vi "Corr Digitizer Save INFO.vi"(7 "path template":path, 8 "error in":errorcluster, 9 "digitizer info":T2, 10 "correction type":T1, 11 "path result":path) -> (0 "error out":errorcluster)   [LabVIEW 2013]
doc: "Saves digitizer/channel INFO file."
uses:
  Corr Digitizer INFO.ctl
  Corr Digitizer INFO item.ctl
  Corr Digitizer INFO parameter.ctl
  Corr CSV Template.ctl
  Corr Digitizer Type.ctl
  octave/infolib.lvlibp/Private/Add key polymorph parts/String.vi
  octave/infolib.lvlibp/Private/Add matrix polymorph parts/1D String.vi
  octave/infolib.lvlibp/Private/Add matrix polymorph parts/2D String.vi
  octave/infolib.lvlibp/Private/Add key polymorph parts/I64.vi
  octave/infolib.lvlibp
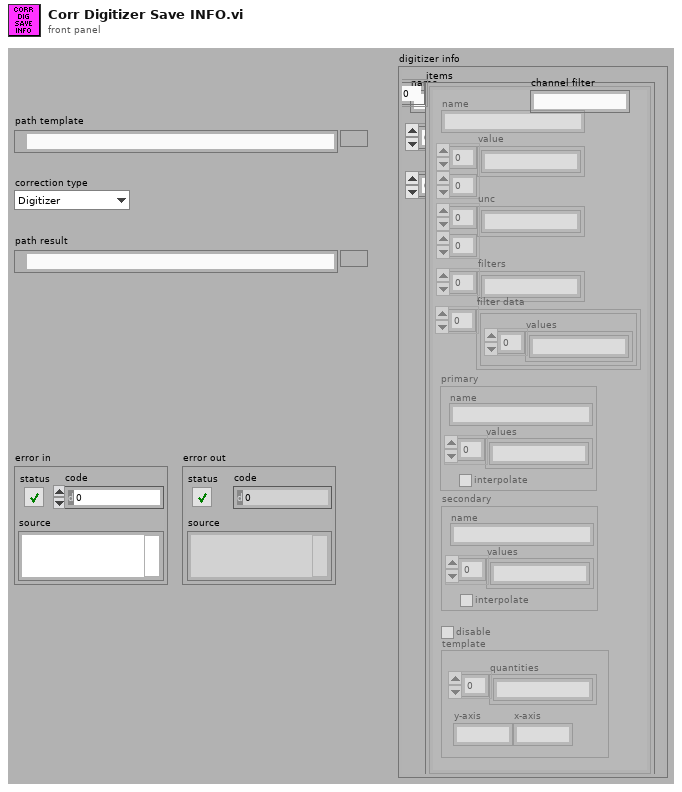
[diagram p1: front panel]
types:
  T1 = typedef "Corr Digitizer Type.ctl" = enum16{"Digitizer", "Channel"}
  T2 = typedef "Corr Digitizer INFO.ctl" = cluster{"name":string, "identifiers":string[], "channel files":string[], "items":T3[], "channel filter":string}
  T3 = typedef "Corr Digitizer INFO item.ctl" = cluster{"name":string, "value":string[][], "unc":string[][], "filters":string[], "primary":T4, "secondary":T4, "filter data":cluster{"values":string[]}[], "disable":bool, "template":T5}
  T4 = typedef "Corr Digitizer INFO parameter.ctl" = cluster{"values":string[], "interpolate":bool, "name":string}
  T5 = typedef "Corr CSV Template.ctl" = cluster{"quantities":string[], "y-axis":string, "x-axis":string}
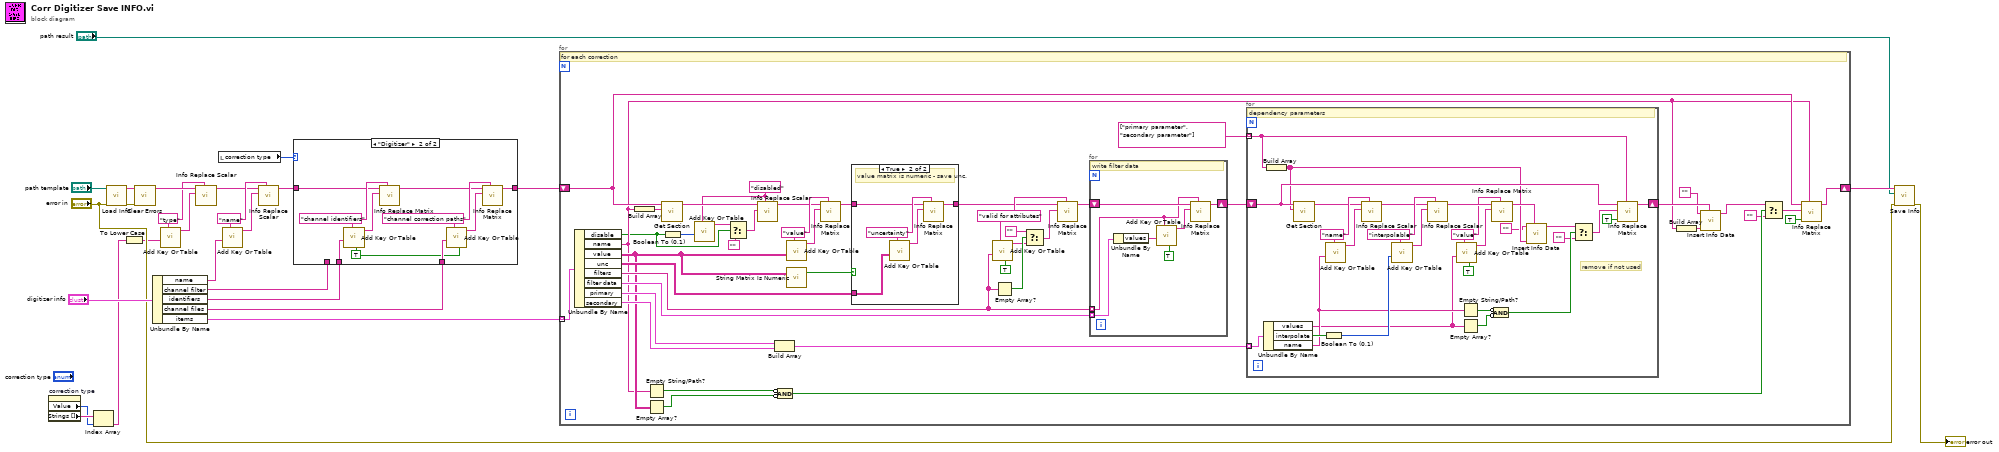
[diagram p0: block diagram]
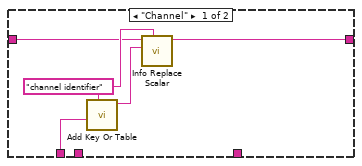
[diagram p3: hidden frame]
diagram:
  w20 = "name" ("key description")
  w21 = "type" ("key description")
  n1 = property on="correction type" class="Enum (strict)"() -> ("Value"=w24:T1, "Strings []"=w25:string[])  [unwired: 2 in, 2 out]
  n2 = Index Array(array=w25, index=w24) -> (element=w8:string)
  n3 = call "Load Info.vi"("error in"="error in", "filename"="path template") -> ("error out"=w2:errorcluster, "info data"=w23:string)  [unwired: 8 in]
  n4 = To Lower Case(string=w8) -> (all lower case string=w1:string)
  n5 = call <vilib>:"Clear Errors.vi"("error in (no error)"=w2) -> ()  [unwired: 6 in, 1 out]
  n6 = Unbundle By Name("digitizer info") -> ("name"=w16:string, "channel filter"=w14:string, "identifiers"=w12:string[], "channel files"=w11:string[], "items"=w10:T3[])
  n7 = call-poly "Add Key Or Table.vi"("key description"=w21, "string"=w1) -> ("info data out"=w22:string)  [unwired: 8 in, 1 out]
  n8 = call "Info Replace Scalar.vi"("key description to replace"=w21, "info data to paste"=w22, "info data in"=w23) -> ("info data out"=w18:string)  [unwired: 8 in]
  n9 = local read "correction type"() -> (w13:T1)
  n10 = call-poly "Add Key Or Table.vi"("key description"=w20, "string"=w16) -> ("info data out"=w19:string)  [unwired: 8 in, 1 out]
  n11 = call "Info Replace Scalar.vi"("key description to replace"=w20, "info data to paste"=w19, "info data in"=w18) -> ("info data out"=w15:string)  [unwired: 8 in]
  n12 = case shown="\"Digitizer\"" w13 {
    tunnel: w15 -> [w28 w38]
    tunnel: w14 -> [w27 _]
    tunnel: [w26 w32] -> w9
    tunnel: w12 -> [_ w37]
    tunnel: w11 -> [_ w33]
    frame "Channel" {
      w29 = "channel identifier" ("key description")
      n13 = call-poly "Add Key Or Table.vi"("key description"=w29, "string"=w27) -> ("info data out"=w30:string)  [unwired: 8 in, 1 out]
      n14 = call "Info Replace Scalar.vi"("key description to replace"=w29, "info data to paste"=w30, "info data in"=w28) -> ("info data out"=w26:string)  [unwired: 8 in]
    }
    frame "Digitizer" {
      w31 = TRUE ("column vector (F)")
      w36 = "channel correction paths" ("key description")
      w39 = "channel identifiers" ("key description")
      n15 = call-poly "Add Key Or Table.vi"("column vector (F)"=w31, "key description"=w39, "string"=w37) -> ("info data out"=w40:string)  [unwired: 7 in, 1 out]
      n16 = call "Info Replace Matrix.vi"("key description to replace"=w39, "info data to paste"=w40, "info data in"=w38) -> ("info data out"=w34:string)  [unwired: 8 in]
      n17 = call-poly "Add Key Or Table.vi"("column vector (F)"=w31, "key description"=w36, "string"=w33) -> ("info data out"=w35:string)  [unwired: 7 in, 1 out]
      n18 = call "Info Replace Matrix.vi"("key description to replace"=w36, "info data to paste"=w35, "info data in"=w34) -> ("info data out"=w32:string)  [unwired: 8 in]
    }
  }
  n19 = for {
    tunnel: w10 -> [w84] mode=indexing
    shift-right: [w54] -> w7
    shift-left: w9 -> [w55]
    w45 = "disabled" ("key description to replace")
    w77 = "valid for attributes" ("key description")
    w81 = "value" ("key description")
    # "for each correction"
    n20 = Unbundle By Name(w84) -> ("disable"=w44:bool, "name"=w52:string, "value"=w62:string[][], "unc"=w78:string[][], "filters"=w68:string[], "filter data"=w70:cluster{"values":string[]}[], "primary"=w66:T4, "secondary"=w65:T4)
    n21 = Build Array(w52) -> (w83:string[])
    n22 = Empty String/Path?(string/path=w52) -> (empty?=w61:bool)
    n23 = Empty Array?(array=w62) -> (empty?=w60:bool)
    n24 = call "Get Section.vi"("sections"=w83, "info data"=w55) -> ("section part"=w48:string)  [unwired: 8 in, 1 out]
    n25 = Boolean To (0,1)(Boolean=w44) -> (0, 1=w46:i16)
    n26 = call-poly "Add Key Or Table.vi"("key description"=w45, "numeric"=w46) -> ("info data out"=w43:string)  [unwired: 8 in, 1 out]
    n27 = Select(t=w43, s=w44, f="") -> (s? t:f=w42:string)
    n28 = call "Info Replace Scalar.vi"("key description to replace"=w45, "info data to paste"=w42, "info data in"=w48) -> ("info data out"=w47:string)  [unwired: 8 in]
    n29 = Build Array(w66, w65) -> (w64:T4[])
    n30 = Compound Arithmetic op=AND(invert w61, invert w60) -> (w59:bool)
    n31 = call-poly "Add Key Or Table.vi"("key description"=w81, "string"=w62) -> ("info data out"=w82:string)  [unwired: 8 in, 1 out]
    n32 = call "String Matrix Is Numeric.vi"("string matrix"=w62) -> ("is numeric"=w80:bool)  [unwired: 1 in, 1 out]
    n33 = call "Info Replace Matrix.vi"("key description to replace"=w81, "info data to paste"=w82, "info data in"=w47) -> ("info data out"=w79:string)  [unwired: 8 in]
    n34 = case shown="True" w80 {
      tunnel: w79 -> [w120 w123]
      tunnel: w78 -> [_ w122]
      tunnel: [w120 w121] -> w76
      frame False {
        # "value is text - no uncertainty\ndata are CSV files"
      }
      frame True {
        w125 = "uncertainty" ("key description")
        # "value matrix is numeric - save unc."
        n35 = call-poly "Add Key Or Table.vi"("key description"=w125, "string"=w122) -> ("info data out"=w124:string)  [unwired: 8 in, 1 out]
        n36 = call "Info Replace Matrix.vi"("key description to replace"=w125, "info data to paste"=w124, "info data in"=w123) -> ("info data out"=w121:string)  [unwired: 8 in]
      }
    }
    n37 = call-poly "Add Key Or Table.vi"("column vector (F)"=TRUE, "key description"=w77, "string"=w68) -> ("info data out"=w73:string)  [unwired: 7 in, 1 out]
    n38 = Empty Array?(array=w68) -> (empty?=w74:bool)
    n39 = Select(t="", s=w74, f=w73) -> (s? t:f=w72:string)
    n40 = call "Info Replace Matrix.vi"("key description to replace"=w77, "info data to paste"=w72, "info data in"=w76) -> ("info data out"=w69:string)  [unwired: 8 in]
    n41 = for {
      tunnel: w70 -> [w117] mode=indexing
      shift-right: [w113] -> w63
      shift-left: w69 -> [w118]
      tunnel: w68 -> [w116] mode=indexing
      # "write filter data"
      n42 = Unbundle By Name(w117) -> ("values"=w115:string[])
      n43 = call-poly "Add Key Or Table.vi"("column vector (F)"=TRUE, "key description"=w116, "string"=w115) -> ("info data out"=w119:string)  [unwired: 7 in, 1 out]
      n44 = call "Info Replace Matrix.vi"("key description to replace"=w116, "info data to paste"=w119, "info data in"=w118) -> ("info data out"=w113:string)  [unwired: 8 in]
    }
    n45 = for {
      tunnel: string[] ["primary parameter", "secondary parameter"] -> [w91] mode=indexing
      tunnel: w64 -> [w109] mode=indexing
      shift-right: [w89] -> w53
      shift-left: w63 -> [w95]
      w100 = "value" ("key description")
      w107 = "interpolable" ("key description")
      w112 = "name" ("key description")
      # "remove if not used"
      # "dependency parameters"
      n46 = Unbundle By Name(w109) -> ("values"=w98:string[], "interpolate"=w105:bool, "name"=w99:string)
      n47 = Build Array(w91) -> (w87:string[])
      n48 = call "Get Section.vi"("sections"=w87, "info data"=w95) -> ("section part"=w110:string)  [unwired: 8 in, 1 out]
      n49 = Boolean To (0,1)(Boolean=w105) -> (0, 1=w104:i16)
      n50 = call-poly "Add Key Or Table.vi"("key description"=w112, "string"=w99) -> ("info data out"=w111:string)  [unwired: 8 in, 1 out]
      n51 = call "Info Replace Scalar.vi"("key description to replace"=w112, "info data to paste"=w111, "info data in"=w110) -> ("info data out"=w106:string)  [unwired: 8 in]
      n52 = call-poly "Add Key Or Table.vi"("key description"=w107, "numeric"=w104) -> ("info data out"=w108:string)  [unwired: 8 in, 1 out]
      n53 = call "Info Replace Scalar.vi"("key description to replace"=w107, "info data to paste"=w108, "info data in"=w106) -> ("info data out"=w102:string)  [unwired: 8 in]
      n54 = call-poly "Add Key Or Table.vi"("column vector (F)"=TRUE, "key description"=w100, "string"=w98) -> ("info data out"=w103:string)  [unwired: 7 in, 1 out]
      n55 = Empty String/Path?(string/path=w99) -> (empty?=w97:bool)
      n56 = Empty Array?(array=w98) -> (empty?=w96:bool)
      n57 = call "Info Replace Matrix.vi"("key description to replace"=w100, "info data to paste"=w103, "info data in"=w102) -> ("info data out"=w88:string)  [unwired: 8 in]
      n58 = Compound Arithmetic op=AND(invert w97, invert w96) -> (w94:bool)
      n59 = call "Insert Info Data.vi"("info data to insert"=w88, "sections"=w87, "info data"="") -> ("info data out"=w86:string)  [unwired: 7 in, 1 out]
      n60 = Select(t=w86, s=w94, f="") -> (s? t:f=w92:string)
      n61 = call "Info Replace Matrix.vi"("key description to replace"=w91, "Is Section (False)"=TRUE, "info data to paste"=w92, "info data in"=w95) -> ("info data out"=w89:string)  [unwired: 7 in]
    }
    n62 = Build Array(w52) -> (w51:string[])
    n63 = call "Insert Info Data.vi"("info data to insert"=w53, "sections"=w51, "info data"="") -> ("info data out"=w50:string)  [unwired: 7 in, 1 out]
    n64 = Select(t=w50, s=w59, f="") -> (s? t:f=w56:string)
    n65 = call "Info Replace Matrix.vi"("key description to replace"=w52, "Is Section (False)"=TRUE, "info data to paste"=w56, "info data in"=w55) -> ("info data out"=w54:string)  [unwired: 7 in]
  }
  n66 = call "Save Info.vi"("error in"="error in", "filename"="path result", "info data"=w7) -> ("error out"=→"error out":errorcluster)  [unwired: 8 in]
